vi "Configure Periodic Random Noise.vi"(0 "template configuration":refnum<class "SV Signal.lvclass">, 7 "level":dbl=1.0, 9 "seed":i32=-1, 11 "error in (no error)":errorcluster) -> (4 "signal configuration":refnum<class "SV Noise.lvclass">, 15 "error out":errorcluster)   [LabVIEW 2017, in "SV Noise.lvclass"]
doc: "Configures a user-defined test signal. Wire the outputs to SV Signal (waveform) VI to generate the test signal, or wire to SV Signal Property Node to configure additional parameters before wiring to the SV Signal (waveform) VI."
uses:
  <vilib>/addons/_NISVFA/_Generation/Signal Generation/SV Noise/SV Noise.lvclass
  C:/Program Files (x86)/National Instruments/LabVIEW 2017/vi.lib/addons/_NISVFA/_Generation/Signal Generation/SV Signal/SV Signal.lvclass
  <vilib>/addons/_NISVFA/_Generation/Signal Generation/SV Signal/SV Signal.lvclass
  <vilib>/addons/_NISVFA/_Generation/Signal Generation/SV Noise/SV Noise.lvclass/SV Noise.ctl
  <vilib>/addons/_NISVFA/_Generation/Signal Generation/SV Signal/Write Post-Measurement Settling Duration.vi
  <vilib>/addons/_NISVFA/_Generation/Signal Generation/SV Signal/Write Pre-Measurement Settling Duration.vi
  <vilib>/addons/_NISVFA/_Generation/Signal Generation/SV Signal/Write Measurement Duration.vi
  <vilib>/addons/_NISVFA/_Generation/Signal Generation/SV Signal/Write Sample Rate.vi
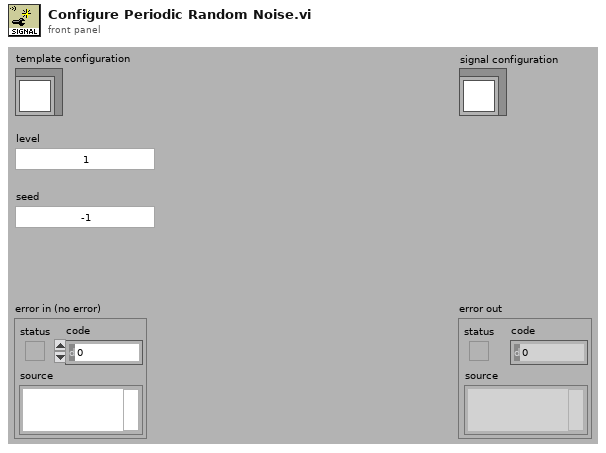
[diagram p1: front panel]
types:
  T1 = enum16{"White noise", "Pink noise", "Periodic random noise"}
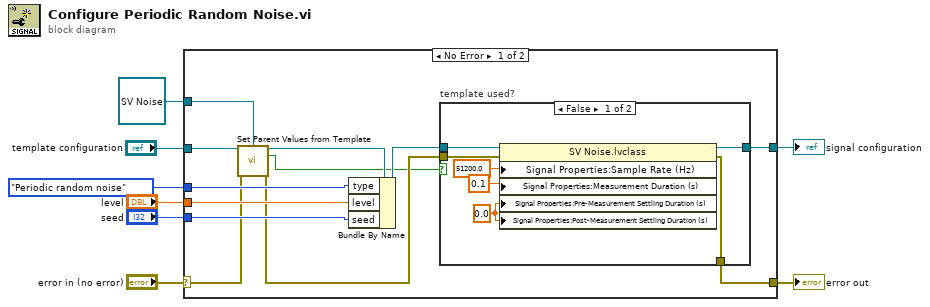
[diagram p0: block diagram]
diagram:
  n1 = case shown="No Error" "error in (no error)" {
    selector: "error in (no error)" -> [w11 w30]
    tunnel: [w15 w30] -> w7
    tunnel: [w16 w31] -> w3
    tunnel: refnum<class "SV Noise.lvclass"> refnum ("BroadbandNoise in") -> [w13 w31]
    tunnel: T1."Periodic random noise" ("type") -> [w20 _]
    tunnel: "level" -> [w19 _]
    tunnel: "seed" -> [w18 _]
    tunnel: "template configuration" -> [w14 _]
    frame No Error {
      n2 = call-dynamic "Set Parent Values from Template.vi"("template configuration"=w14, "signal configuration in"=w13, "error in (no error)"=w11) -> ("signal configuration out"=w12:refnum<class "SV Noise.lvclass">, "template used?"=w9:bool, "error out"=w10:errorcluster)  [unwired: 10 in]
      n3 = Bundle By Name(cluster=w12, "type"=w20, "level"=w19, "seed"=w18) -> (w17:refnum<class "SV Noise.lvclass">)
      n4 = case "template used?" shown="False" w9 {
        tunnel: w17 -> [w26 w29]
        tunnel: [w25 w29] -> w16
        tunnel: [w24 w28] -> w15
        tunnel: w10 -> [w21 w28]
        frame False {
          w27 = 0.0 ("settling time_s")
          n5 = property class="SV Noise.lvclass"(reference=w26, error in=w21, "Signal Properties:Sample Rate (Hz)"=51200.0 ("SampleRate_Hz"), "Signal Properties:Measurement Duration (s)"=0.1 ("integration time_s"), "Signal Properties:Pre-Measurement Settling Duration (s)"=w27, "Signal Properties:Post-Measurement Settling Duration (s)"=w27) -> (reference out=w25:refnum<class "SV Noise.lvclass">, error out=w24:errorcluster)
        }
        frame True {
        }
      }
    }
    frame Error {
    }
  }
  "error out" <- w7
  "signal configuration" <- w3
